vi "KalmanFilter_GetXHat.vi"(11 "in KalmanFilter":T2) -> (3 "xHat":T1)   [LabVIEW 2019, in "Trajectory_Library.lvlib"]
doc: "Returns the state estimate x-hat.\n \nInputs:\n - KalmanFilter -- filter data cluster\n\nOutputs:\n - xHat - The state estimate x-hat."
uses:
  Trajectory_Library.lvlib
  KALMAN_FILTER.ctl
  <vilib>/Analysis/Matrix/Datatypes/RealMatrix.ctl
  LINEAR_SYSTEM.ctl
  <vilib>/Analysis/Matrix/NI_Matrix.lvlib
panel:
  # "Steady State Gain  \n<States,Outputs>"
  # "State Estimate <Statess,1>"
  # "<States,States>"
  # "<States,Inputs>"
  # "<Outputs,States>"
  # "<Outputs,Inputs>"
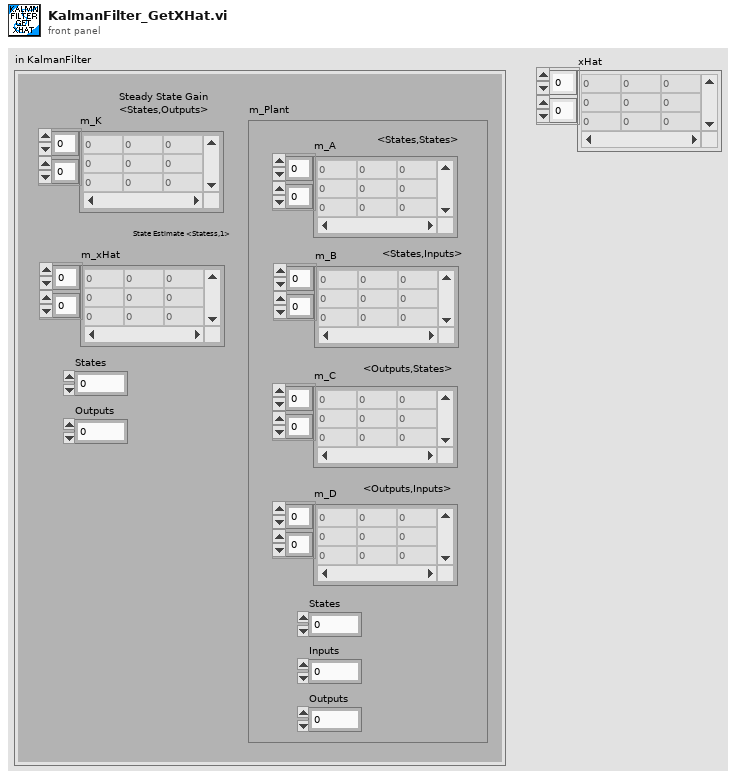
[diagram p1: front panel]
types:
  T1 = typedef "NI_Matrix.lvlib/RealMatrix.ctl" = dbl[][]
  T2 = typedef "Trajectory_Library.lvlib/KALMAN_FILTER.ctl" = cluster{"m_K":T1, "m_xHat":T1, "States":i32, "Outputs":i32, "m_Plant":T3}
  T3 = typedef "Trajectory_Library.lvlib/LINEAR_SYSTEM.ctl" = cluster{"m_A":T1, "m_B":T1, "m_C":T1, "m_D":T1, "States":i32, "Inputs":i32, "Outputs":i32}
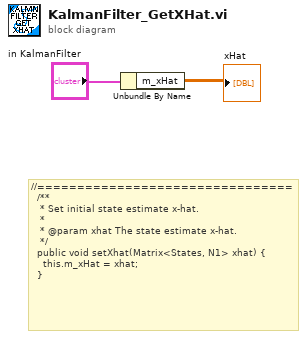
[diagram p0: block diagram]
diagram:
  # "//================================\n  /**\n   * Set initial state estimate x-hat.\n   *\n   * @param xhat The state estimate x-hat.\n   */\n  public void setXhat(Matrix<States, N1> xhat) {\n    this.m_xHat = xhat;\n  }"
  n1 = Unbundle By Name("in KalmanFilter") -> ("m_xHat"=→"xHat":T1)
